vi "user process.vi"(8 "error in":errorcluster, 10 "Parameters to process":T2, 11 "State Machine runtime in":refnum<class "State Machine runtime.lvclass">) -> (0 "error out":errorcluster, 2 "Results from processing":T1, 3 "State Machine runtime out":refnum<class "State Machine runtime.lvclass">)   [LabVIEW 2021, in "State Machine runtime.lvclass"]
uses:
  State Machine runtime.lvclass
  parameter user data.ctl
  result user data.ctl
  State Machine runtime.lvclass/State Machine runtime.ctl
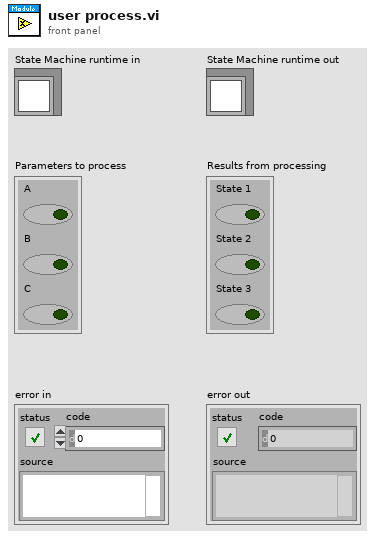
[diagram p1: front panel]
types:
  T1 = typedef "State Machine runtime.lvclass/result user data.ctl" = cluster{"State 1":bool, "State 2":bool, "State 3":bool}
  T2 = typedef "State Machine runtime.lvclass/parameter user data.ctl" = cluster{"A":bool, "B":bool, "C":bool}
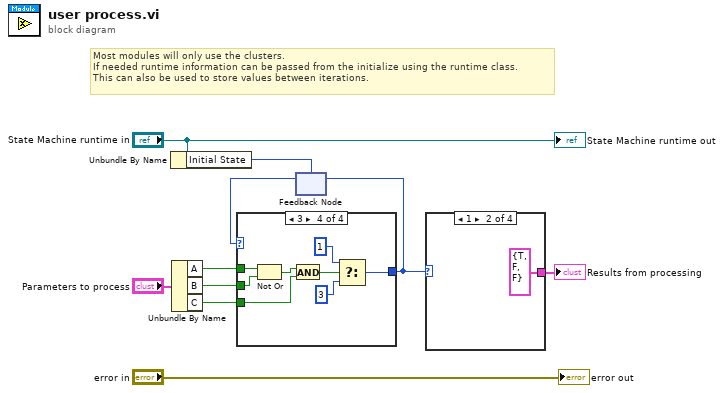
[diagram p0: block diagram]
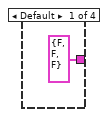
[diagram p2: hidden frame]
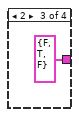
[diagram p3: hidden frame]
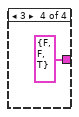
[diagram p4: hidden frame]
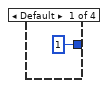
[diagram p5: hidden frame]
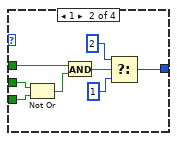
[diagram p6: hidden frame]
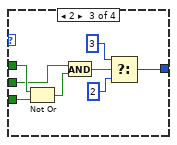
[diagram p7: hidden frame]
diagram:
  # "Most modules will only use the clusters.\nIf needed runtime information can be passed from the initialize using the runtime class.\nThis can also be used to store values between iterations."
  n1 = Unbundle By Name("State Machine runtime in") -> ("Initial State"=w6:i32)
  n2 = Unbundle By Name("Parameters to process") -> ("A"=w4:bool, "B"=w3:bool, "C"=w2:bool)
  n3 = feedback #1(w6) -> (w5:i32)
  n4 = case shown="3" w5 {
    tunnel: w4 -> [_ w19 w21 w31]
    tunnel: w3 -> [_ w18 w20 w30]
    tunnel: w2 -> [_ w17 w27 w28]
    tunnel: [1 ("Initial State") w12 w22 w32] -> w1
    frame Default {
    }
    frame 1 {
      n5 = Not Or(1:w17, 2:w18) -> (0:w16:bool)
      n6 = And(x=w19, y=w16) -> (x .and. y?=w15:bool)
      n7 = Select(t=2, s=w15, f=1 ("Initial State")) -> (s? t:f=w12:i32)
    }
    frame 2 {
      n8 = Not Or(1:w27, 2:w21) -> (0:w26:bool)
      n9 = And(x=w20, y=w26) -> (x .and. y?=w25:bool)
      n10 = Select(t=3, s=w25, f=2 ("Initial State")) -> (s? t:f=w22:i32)
    }
    frame 3 {
      n11 = Not Or(1:w30, 2:w31) -> (0:w29:bool)
      n12 = And(x=w29, y=w28) -> (x .and. y?=w35:bool)
      n13 = Select(t=1, s=w35, f=3 ("Initial State")) -> (s? t:f=w32:i32)
    }
  }
  n14 = feedback-in #1(w1) -> ()
  n15 = case shown="1" w1 {
    tunnel: [T1 {"State 1"=FALSE, "State 2"=FALSE, "State 3"=FALSE} ("Results from processing") T1 {"State 1"=TRUE, "State 2"=FALSE, "State 3"=FALSE} ("Results from processing") T1 {"State 1"=FALSE, "State 2"=TRUE, "State 3"=FALSE} ("Results from processing") T1 {"State 1"=FALSE, "State 2"=FALSE, "State 3"=TRUE} ("Results from processing")] -> w7
    frame Default {
    }
    frame 1 {
    }
    frame 2 {
    }
    frame 3 {
    }
  }
  "Results from processing" <- w7
  "error out" <- "error in"
  "State Machine runtime out" <- "State Machine runtime in"
